vi "Set Port Status.vi"(8 "error in (no error)":errorcluster, 9 "Value":string, 10 "Port":dbl, 11 "object in":refnum<class "NXP.lvclass">) -> (0 "error out":errorcluster, 3 "object out":refnum<class "NXP.lvclass">)   [LabVIEW 2020, in "NXP.lvclass"]
uses:
  NXP.lvclass
  NXP.lvclass/NXP.ctl
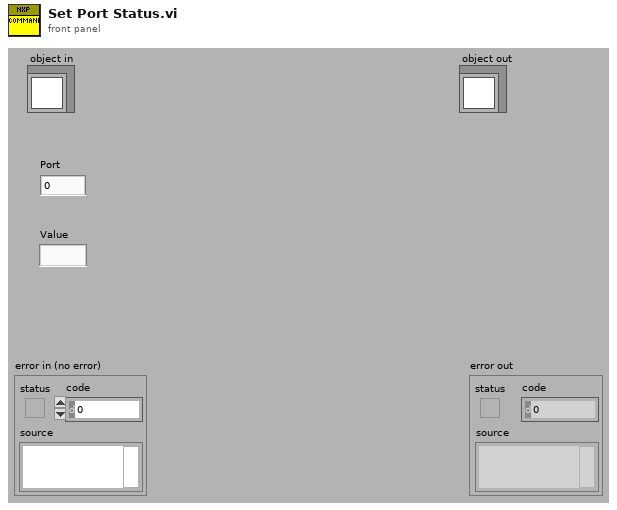
[diagram p1: front panel]
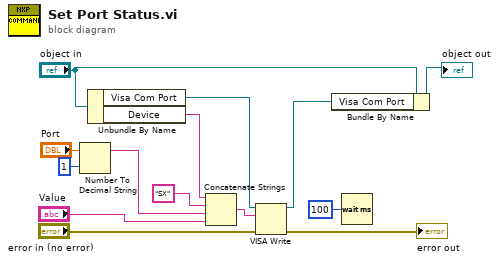
[diagram p0: block diagram]
diagram:
  n1 = Number To Decimal String(number="Port", width (-)=i16 1) -> (decimal integer string=w6:string)
  n2 = Unbundle By Name("object in") -> ("Visa Com Port"=w12:refnum<visa-resource-name>, "Device"=w10:string)
  n3 = Concatenate Strings(w10, "SX" ("string"), w6, "Value") -> (w11:string)
  n4 = VISA Write(VISA resource name=w12, write buffer=w11, error in (no error)="error in (no error)") -> (VISA resource name out=w2:refnum<visa-resource-name>, error out=→"error out":errorcluster)  [unwired: 1 out]
  n5 = Bundle By Name(cluster="object in", "Visa Com Port"=w2) -> (→"object out":refnum<class "NXP.lvclass">)
  n6 = Wait (ms)(milliseconds to wait=u32 100) -> ()  [unwired: 1 out]
